vi "OXITC503 _Config_ Basic Configuration and Sweep Stages Setup.vi"(0 "VISA session in":refnum<visa-resource-name>="GPIB::2", 1 "Basic Parameters":T1={"Set Point (K)"=0.0, "temp P"=80.0, "temp I"=70.0, "temp D"=60.0} {"temp D" min=0 max=99 format="%.2f"; "temp I" min=0 max=99 format="%.2f"; "temp P" min=0 max=99 format="%.2f"; "Set Point (K)" format="%.2f"}, 2 "Auto Status":T3(ring)=enum."Heater and Gas Auto", 3 "Auto PID (Off)":enum16{"Auto PID Off", "Auto PID On"}(ring), 4 "Controlling Sensor":u16(ring) items=["Sensor 1", "Sensor 2", "Sensor 3"], 5 "error in":errorcluster, 6 "Heater Output (%)":dbl format="%.2f", 7 "Edit Sweep Stages?":bool, 8 "Gas Valve (%)":dbl format="%.2f", 9 "New Sweep Stages (temp.)":T2(array[cluster]) {"Hold Time For Stage" min=0.0 max=1339.9 step=0.1 format="%.2f"; "Sweep Time for Stage" min=0.0 max=1339.9 step=0.1 format="%.2f"; "Set Point" format="%.2f"}, 11 "Start Sweep after setup? (Off)":enum16{"Sweep Off", "Sweep On"}(ring)) -> (14 "VISA session out":refnum<visa-resource-name>, 19 "error out":errorcluster)   [LabVIEW 2013]
doc: "Setups ITC503, allows the user to configure the Swep stages. Does not edit the AUTO-PID table.\n\nNotes:\n\n- If there is a running Sweep it will be stopped.\n- Heater Output (Gas Valve) is only used if the ITC is in HEATER (GAS) AUTO mode."
panel:
  # "Basic Setup (temp.)"
  # "FOR MANUAL HEATER"
  # "FOR MANUAL GAS"
  # "Advanced"
  # "Program Complete Sweep\n(Only For Sweeps)"
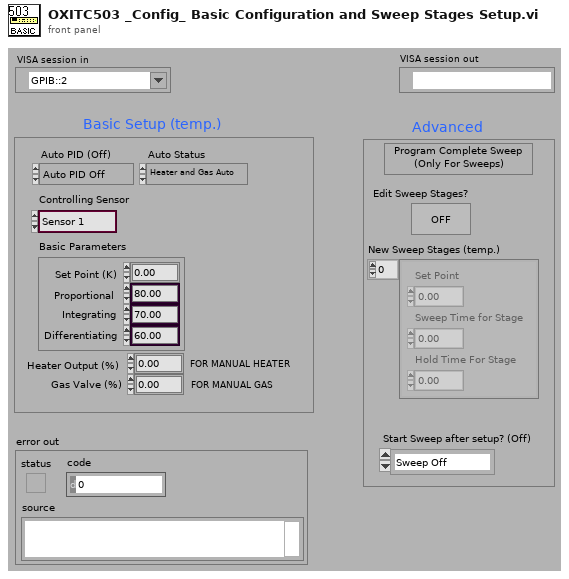
[diagram p1: front panel]
types:
  T1 = cluster{"Set Point (K)":dbl, "temp P":sgl, "temp I":sgl, "temp D":sgl}
  T2 = cluster{"Set Point":dbl, "Sweep Time for Stage":dbl, "Hold Time For Stage":dbl}[]
  T3 = enum16{"Heater and gas Manual", "Heater Auto, Gas Manual", "Heater Manual, Gas Auto", "Heater and Gas Auto"}
  T4 = cluster{"Setpoint":dbl, "Control Sensor":enum16{"Sensor 1", "Sensor 2", "Sensor 3"}, "P":dbl, "I":dbl, "D":dbl}
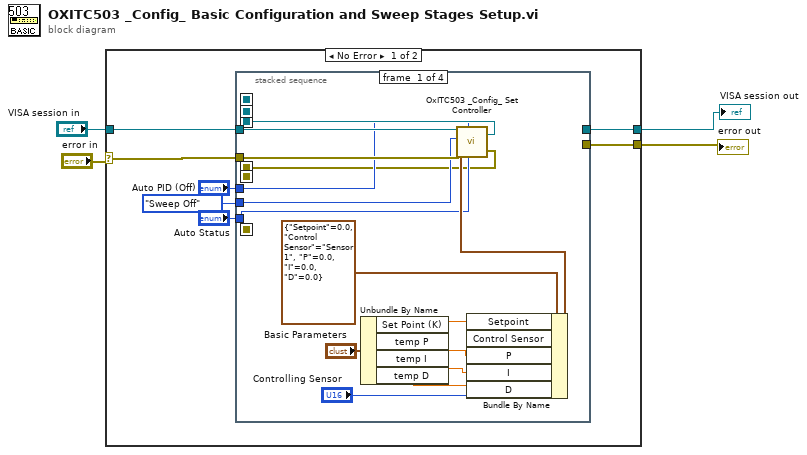
[diagram p0: block diagram]
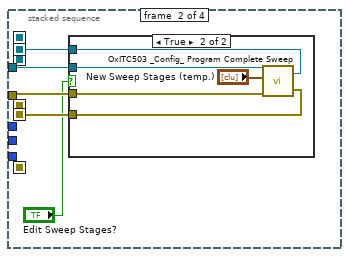
[diagram p2: hidden frame]
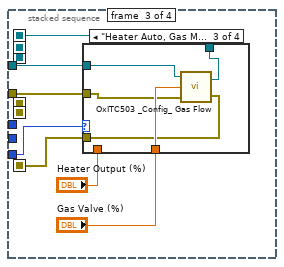
[diagram p4: hidden frame]
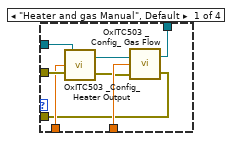
[diagram p5: hidden frame]
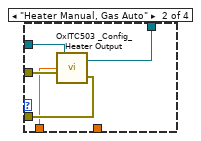
[diagram p6: hidden frame]
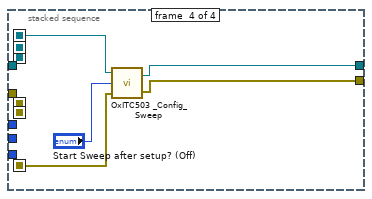
[diagram p8: hidden frame]
diagram:
  n1 = case shown="No Error" "error in" {
    selector: "error in" -> [w11 w72]
    tunnel: [w5 w72] -> w4
    tunnel: [w6 w71] -> w3
    tunnel: "VISA session in" -> [w10 w71]
    frame No Error {
      n2 = stacked-sequence {
        seq-local: [w16 _ _ _] -> [_ _ _ _]
        seq-local: [w12 _ _ _] -> [_ _ _ _]
        seq-local: [_ w29 _ _] -> [_ _ _ _]
        seq-local: [_ w28 _ _] -> [_ _ _ _]
        seq-local: [_ _ w39 _] -> [_ _ _ w70]
        seq-local: [_ _ w42 _] -> [_ _ _ w69]
        tunnel: w10 -> [w23 w31 w43 _]
        tunnel: w11 -> [w22 w30 w44 _]
        tunnel: "Auto PID (Off)" -> [w15 _ _ _]
        tunnel: enum16{"Sweep Off", "Sweep On"}."Sweep Off" ("Start Sweep after setup? (Off)") -> [w14 _ _ _]
        tunnel: "Auto Status" -> [w13 _ w45 _]
        tunnel: [_ _ _ w67] -> w6
        tunnel: [_ _ _ w66] -> w5
        frame #0 {
          n3 = Unbundle By Name("Basic Parameters") -> ("Set Point (K)"=w17:dbl, "temp P"=w20:sgl, "temp I"=w19:sgl, "temp D"=w18:sgl)
          n4 = Bundle By Name(cluster=T4 {"Setpoint"=0.0, "Control Sensor"=enum."Sensor 1", "P"=0.0, "I"=0.0, "D"=0.0} ("Temperature Control Settings"), "Setpoint"=w17, "Control Sensor"="Controlling Sensor", "P"=w20, "I"=w19, "D"=w18) -> (w24:T4)
          n5 = call "OxITC503 _Config_ Set Controller.vi"("Auto Status"=w13, "Auto PID (Off)"=w15, "error in (no error)"=w22, "Temperature Control Settings"=w24, "Sweep Status (Off)"=w14, "VISA session"=w23) -> ("error out"=w12:errorcluster, "VISA session"=w16:refnum<visa-resource-name>)
        }
        frame #1 {
          n6 = case shown="True" "Edit Sweep Stages?" {
            tunnel: w31 -> [w33 w38]
            tunnel: w30 -> [w32 w37]
            tunnel: [w33 w35] -> w29
            tunnel: [w32 w34] -> w28
            frame False {
            }
            frame True {
              n7 = call "OxITC503 _Config_ Program Complete Sweep.vi"("error in (no error)"=w37, "Sweep Program"="New Sweep Stages (temp.)", "VISA session"=w38) -> ("error out"=w34:errorcluster, "VISA session"=w35:refnum<visa-resource-name>)  [unwired: 3 in]
            }
          }
        }
        frame #2 {
          n8 = case shown="\"Heater and gas Manual\", Default" w45 {
            tunnel: w43 -> [w53 w58 w62 w64]
            tunnel: w44 -> [w52 w57 w61 w65]
            tunnel: [w46 w56 w60 w65] -> w42
            tunnel: "Heater Output (%)" -> [w51 w55 _ _]
            tunnel: "Gas Valve (%)" -> [w50 _ w63 _]
            tunnel: [w47 w54 w59 w64] -> w39
            frame "Heater and gas Manual", Default {
              n9 = call "OxITC503 _Config_ Heater Output.vi"("error in"=w52, "Heater Output (%)"=w51, "VISA session"=w53) -> ("error out (no error)"=w49:errorcluster, "VISA session"=w48:refnum<visa-resource-name>)
              n10 = call "OxITC503 _Config_ Gas Flow.vi"("error in"=w49, "Gas Flow Value"=w50, "VISA session"=w48) -> ("error out (no error)"=w46:errorcluster, "VISA session"=w47:refnum<visa-resource-name>)
            }
            frame "Heater Manual, Gas Auto" {
              n11 = call "OxITC503 _Config_ Heater Output.vi"("error in"=w57, "Heater Output (%)"=w55, "VISA session"=w58) -> ("error out (no error)"=w56:errorcluster, "VISA session"=w54:refnum<visa-resource-name>)
            }
            frame "Heater Auto, Gas Manual" {
              n12 = call "OxITC503 _Config_ Gas Flow.vi"("error in"=w61, "Gas Flow Value"=w63, "VISA session"=w62) -> ("error out (no error)"=w60:errorcluster, "VISA session"=w59:refnum<visa-resource-name>)
            }
            frame "Heater and Gas Auto" {
            }
          }
        }
        frame #3 {
          n13 = call "OxITC503 _Config_ Sweep.vi"("error in"=w69, "Sweep Status"="Start Sweep after setup? (Off)", "VISA session"=w70) -> ("error out (no error)"=w66:errorcluster, "VISA session"=w67:refnum<visa-resource-name>)
        }
      }
    }
    frame Error {
    }
  }
  "error out" <- w4
  "VISA session out" <- w3
